vi "make_plot_main.vi"(4 "Graph Scale By":T5, 7 "Plot Property":T6={"Projection Properties"={"Draw XY"=FALSE, "Draw YZ"=FALSE, "Draw XZ"=FALSE}, "Surface Properties"={"Draw surface"=TRUE, "Opacity"=100.0, "Shading"=TRUE, "Specular"=100, "Color Map"=[], "Interpolate Color"=TRUE, "Absolute Colormap"=TRUE}, "Contour Properties"={"Contour color"=0, "Axis"=enum."X", "Draw contour"=FALSE, "Antialias"=FALSE, "Line Width"=0.0, "Contour Line Style"=enum."Solid", "Mode"=enum."Levels", "Levels"=5.0, "Intervals"=1.0, "Anchored At"=0.0, "Anchored"=FALSE, "Level List"=[]}, "Normal Properties"={"Normal color"=0, "Normal Length"=0.0, "Normal Width"=0.0, "Draw Normal"=FALSE, "Antialiasing"=FALSE}, "Points/Lines Properties"={"Color"=0, "Antialiasing"=FALSE, "Point Size"=0.0, "Points / Lines"=enum."None", "Point Style"=enum."Point", "Line Style"=enum."Solid", "Line Width"=0.0}, "Plot ID"=0, "Coordinate System"=enum."Cartesian"}, 8 "Graph Range Min/Max":T2, 9 "Plot Representation":T1, 10 "PL Transformation":sgl[][](array[numeric])) -> (1 "PL Scene Object Out":refnum<vi>, 2 "Surface Mesh Out":refnum<vi>, 3 "Plot Scene Object Out":refnum<vi>)   [LabVIEW 2020, in "3DPC_SurfacePlot.xctl"]
uses:
  <vilib>/Native 3D Graph/xcontrol/3DPC_SurfacePlot.xctl
  <vilib>/Native 3D Graph/typedefs/prop_plot_all.ctl
  <vilib>/Native 3D Graph/typedefs/prop_plot_projection.ctl
  <vilib>/Native 3D Graph/typedefs/prop_plot_surface.ctl
  <vilib>/Native 3D Graph/typedefs/prop_plot_contour.ctl
  <vilib>/Native 3D Graph/typedefs/prop_plot_normal.ctl
  <vilib>/Native 3D Graph/typedefs/prop_plot_point_line.ctl
  <vilib>/Native 3D Graph/typedefs/range_cluster.ctl
  <vilib>/Native 3D Graph/typedefs/min_max.ctl
  <vilib>/Native 3D Graph/typedefs/vector.ctl
  <vilib>/Native 3D Graph/typedefs/plot_rep.ctl
  <vilib>/Native 3D Graph/typedefs/plot_rep_mesh_data.ctl
  <vilib>/picture/3D Picture Control/Object/Create Object (name).vi
  <vilib>/picture/3D Picture Control/NI_3D Picture Control.lvlib
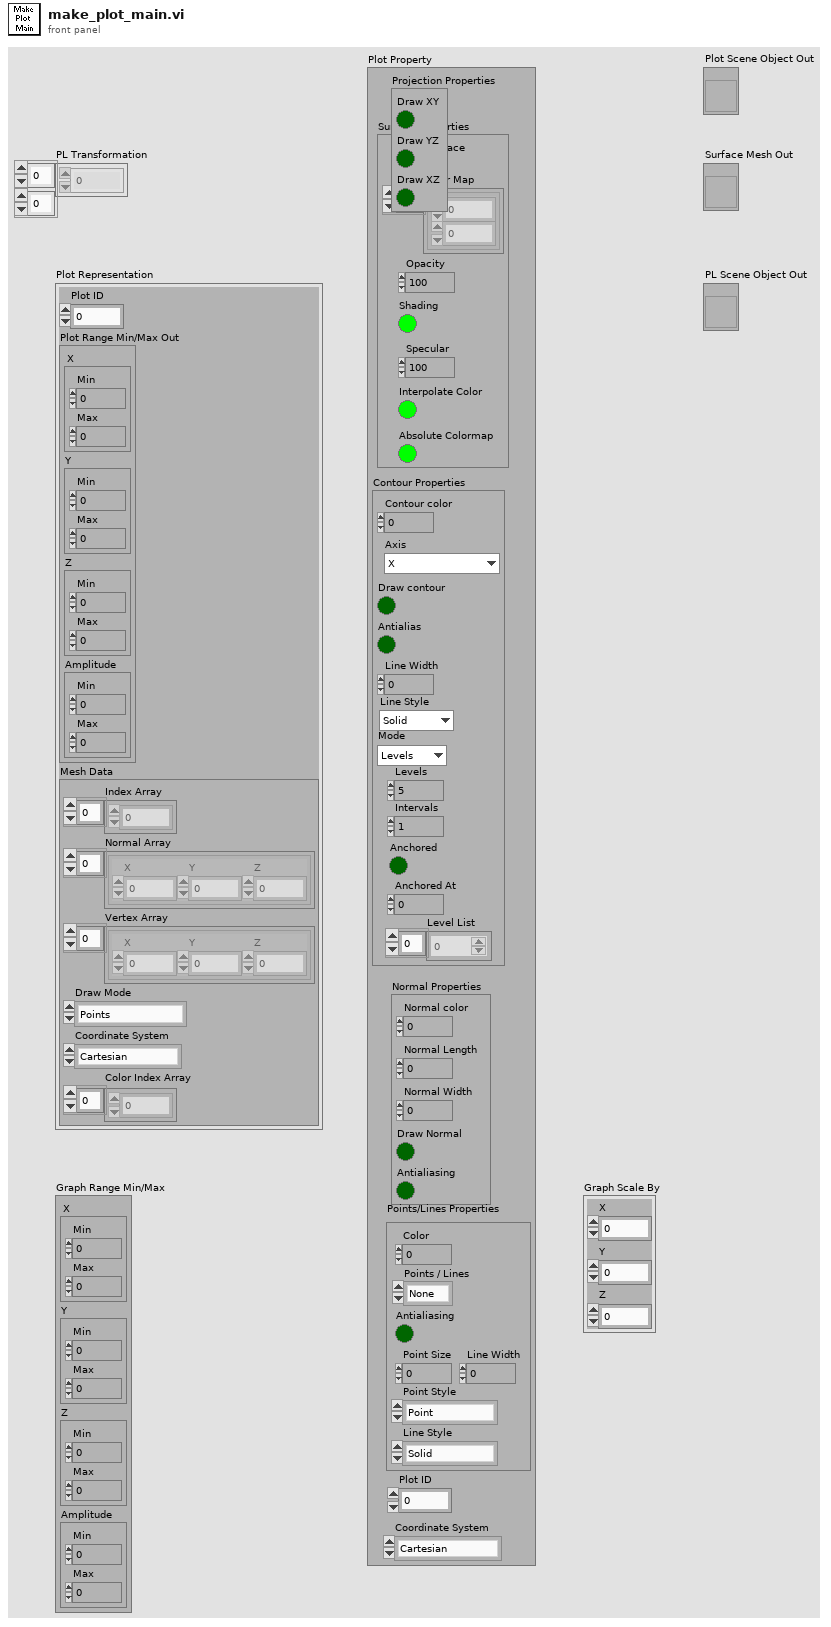
[diagram p1: front panel]
types:
  T1 = typedef "3DPC_SurfacePlot.xctl/plot_rep.ctl" = cluster{"Plot ID":i32, "Plot Range Min/Max Out":T2, "Mesh Data":T4}
  T2 = typedef "3DPC_SurfacePlot.xctl/range_cluster.ctl" = cluster{"X":T3, "Y":T3, "Z":T3, "Amplitude":T3}
  T3 = typedef "3DPC_SurfacePlot.xctl/min_max.ctl" = cluster{"Min":sgl, "Max":sgl}
  T4 = typedef "3DPC_SurfacePlot.xctl/plot_rep_mesh_data.ctl" = cluster{"Index Array":u32[], "Normal Array":cluster{"X":sgl, "Y":sgl, "Z":sgl}[], "Vertex Array":cluster{"X":sgl, "Y":sgl, "Z":sgl}[], "Draw Mode":enum16{"Points", "Lines", "Line Strip", "Line Loop", "Triangles", "Triangle Strip", "Triangle Fan", "Quads", "Quad Strip", "Polygon"}, "Coordinate System":enum16{"Cartesian", "Cylindrical", "Spherical"}, "Color Index Array":i32[]}
  T5 = typedef "3DPC_SurfacePlot.xctl/vector.ctl" = cluster{"X":sgl, "Y":sgl, "Z":sgl}
  T6 = typedef "3DPC_SurfacePlot.xctl/prop_plot_all.ctl" = cluster{"Projection Properties":T7, "Surface Properties":T8, "Contour Properties":T9, "Normal Properties":T10, "Points/Lines Properties":T11, "Plot ID":i32, "Coordinate System":enum16{"Cartesian", "Cylindrical", "Spherical"}}
  T7 = typedef "3DPC_SurfacePlot.xctl/prop_plot_projection.ctl" = cluster{"Draw XY":bool, "Draw YZ":bool, "Draw XZ":bool}
  T8 = typedef "3DPC_SurfacePlot.xctl/prop_plot_surface.ctl" = cluster{"Draw surface":bool, "Opacity":dbl, "Shading":bool, "Specular":i32, "Color Map":cluster{dbl, u32}[], "Interpolate Color":bool, "Absolute Colormap":bool}
  T9 = typedef "3DPC_SurfacePlot.xctl/prop_plot_contour.ctl" = cluster{"Contour color":u32, "Axis":enum16{"X", "Y", "Z"}, "Draw contour":bool, "Antialias":bool, "Line Width":sgl, "Contour Line Style":enum16{"Solid", "Dash", "Dot", "Dash Dot"}, "Mode":enum16{"Levels", "Intervals", "Level List"}, "Levels":sgl, "Intervals":sgl, "Anchored At":sgl, "Anchored":bool, "Level List":dbl[]}
  T10 = typedef "3DPC_SurfacePlot.xctl/prop_plot_normal.ctl" = cluster{"Normal color":u32, "Normal Length":sgl, "Normal Width":sgl, "Draw Normal":bool, "Antialiasing":bool}
  T11 = typedef "3DPC_SurfacePlot.xctl/prop_plot_point_line.ctl" = cluster{"Color":u32, "Antialiasing":bool, "Point Size":sgl, "Points / Lines":enum16{"None", "Points", "Lines", "Both"}, "Point Style":enum16{"Point", "EmptySquare", "Asterisk", "Diamond", "EmptyCircle", "Circle", "X"}, "Line Style":enum16{"Solid", "Dash", "Dot", "Dash Dot"}, "Line Width":sgl}
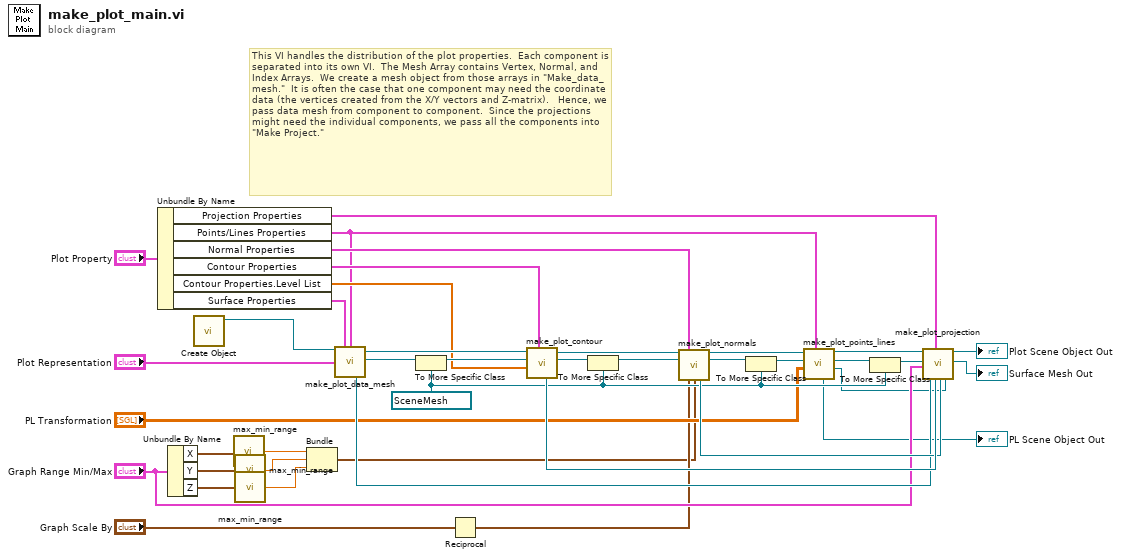
[diagram p0: block diagram]
diagram:
  w18 = refnum<vi> refnum ("Surface Mesh Refnum")
  # "This VI handles the distribution of the plot properties.  Each component is separated into its own VI.  The Mesh Array contains Vertex, Normal, and Index Arrays.  We create a mesh object from those arrays in \"Make_data_mesh.\"  It is often the case that one component may need the coordinate data (the vertices created from the X/Y vectors and Z-matrix).   Hence, we pass data mesh from component to component.  Since the projections might need the individual components, we pass all the components into \"Make Project.\""
  n1 = Unbundle By Name("Plot Property") -> ("Projection Properties"=w28:T7, "Points/Lines Properties"=w8:T11, "Normal Properties"=w27:T10, "Contour Properties"=w26:T9, "Contour Properties.Level List"=w11:dbl[], "Surface Properties"=w25:T8)
  n2 = Unbundle By Name("Graph Range Min/Max") -> ("X"=w20:T3, "Y"=w19:T3, "Z"=w17:T3)
  n3 = call-poly <vilib>:"Create Object.vi"() -> ("Scene:New Object"=w7:refnum<vi>)  [unwired: 10 in, 1 out]
  n4 = call <vilib>:"max_min_range.vi"("Z Min/Max"=w20) -> ("Range"=w15:sgl)  [unwired: 8 out]
  n5 = call <vilib>:"max_min_range.vi"("Z Min/Max"=w19) -> ("Range"=w14:sgl)  [unwired: 8 out]
  n6 = call <vilib>:"max_min_range.vi"("Z Min/Max"=w17) -> ("Range"=w13:sgl)  [unwired: 8 out]
  n7 = Bundle("Range"=w15, "Range"=w14, "Range"=w13) -> (w2:cluster{"Range":sgl, "Range":sgl, "Range":sgl})  [unwired: 1 out]
  n8 = call <vilib>:"make_plot_data_mesh.vi"("Scene:In Object"=w7, "Surface Properties"=w25, "Points/Lines Properties"=w8, "Plot Representation"="Plot Representation") -> ("Collection Scene Object"=w24:refnum<vi>, "Data Mesh Out"=w23:refnum<vi>, "Data Scene Object Out"=w22:refnum<vi>)  [unwired: 1 in, 8 out]
  n9 = To More Specific Class(target class=w18, reference=w23) -> (specific class reference=w29:refnum<vi>)  [unwired: 1 in, 1 out]
  n10 = Reciprocal(x="Graph Scale By") -> (1/x=w3:T5)
  n11 = call <vilib>:"make_plot_contour.vi"("Contour Properties"=w26, "Contour Array"=w11, "Surface Mesh In"=w29, "Scene Object In"=w24) -> ("Surface Mesh Out"=w40:refnum<vi>, "Collection Scene Object Out"=w38:refnum<vi>, "Contour Scene Object Out"=w32:refnum<vi>)  [unwired: 2 in, 3 out]
  n12 = To More Specific Class(target class=w18, reference=w40) -> (specific class reference=w37:refnum<vi>)  [unwired: 1 in, 1 out]
  n13 = call <vilib>:"make_plot_normals.vi"("Scene Object In"=w38, "Normal Properties"=w27, "Data Mesh In"=w37, "Plot Pre-Scale"=w3, "Graph Pre-Scale"=w2) -> ("Scene Object Out"=w39:refnum<vi>, "Data Mesh Out"=w33:refnum<vi>, "Normal Scene Object Out"=w31:refnum<vi>)  [unwired: 1 in, 7 out]
  n14 = To More Specific Class(target class=w18, reference=w33) -> (specific class reference=w10:refnum<vi>)  [unwired: 1 in, 1 out]
  n15 = call <vilib>:"make_plot_points_lines.vi"("Points/Lines Properties"=w8, "Transformation"="PL Transformation", "Surface Mesh In"=w10, "Plot Scene Object In"=w39) -> ("Unscaled PL"=w4:refnum<vi>, "Drawable"=w35:refnum<vi>, "Plot Scene Object Out"=w36:refnum<vi>, "PL Scene Object Out"=→"PL Scene Object Out":refnum<vi>)  [unwired: 4 out]
  n16 = To More Specific Class(target class=w18, reference=w35) -> (specific class reference=w34:refnum<vi>)  [unwired: 1 in, 1 out]
  n17 = call <vilib>:"make_plot_projection.vi"("Plot Scene Object In"=w36, "Surface Mesh In"=w34, "Minimum"="Graph Range Min/Max", "Data Mesh Object In"=w22, "Projection Properties"=w28, "Contour Object In"=w32, "Normals Object In"=w31, "PL Object In"=w4) -> ("Plot Scene Object Out"=→"Plot Scene Object Out":refnum<vi>, "Surface Mesh Out"=→"Surface Mesh Out":refnum<vi>)  [unwired: 1 in, 9 out]
